vi "parse_int32.vi"   [LabVIEW 2016]
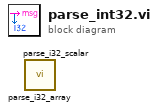
[diagram p0: block diagram]
diagram:
  n1 = call "parse_i32_array.vi"() -> ()  [unwired: 5 in, 3 out]
  n2 = call "parse_i32_scalar.vi"() -> ()  [unwired: 5 in, 3 out]
